vi "celsiustofahrenheit.vi"() -> ()   [LabVIEW 2018]
panel:
  in  "stop":bool
  out "Fahrenheit":dbl
  out "Celsius":dbl
  in  "Slide":dbl(slide) scale=-30.0..50.0
  out "Thermometer":dbl(slide) scale=0.0..150.0
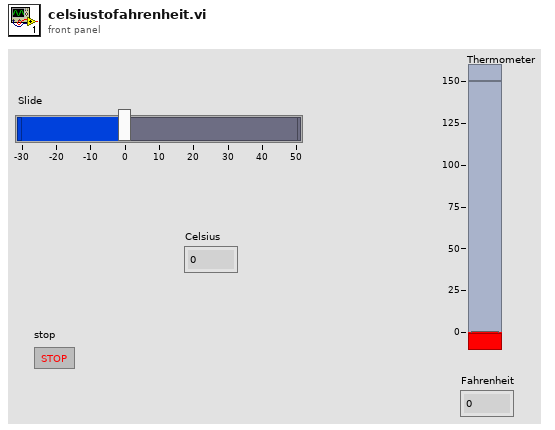
[diagram p1: front panel]
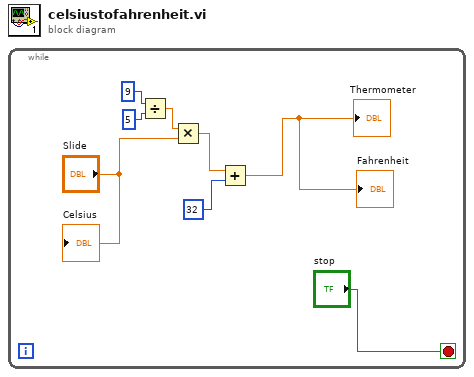
[diagram p0: block diagram]
diagram:
  n1 = while {
    stop <- "stop" stop-if-true
    n2 = Divide(x=9, y=5) -> (x/y=w8:dbl)
    n3 = Multiply(x=w8, y="Slide") -> (x*y=w5:dbl)
    n4 = Add(x=w5, y=32) -> (x+y=→"Thermometer" →"Fahrenheit":dbl)
    "Celsius" <- "Slide"
  }
